vi "Get Line Colour.vi"(8 "Error In":errorcluster, 9 "Session In":T2="cam0") -> (0 "Error Out":errorcluster, 1 "Session Out":T2="cam0", 2 "Confidence (0-100)":dbl=99.96947916666667, 3 "Colour":T3=enum."None", 5 "Blue":dbl=0.030520833333333334)   [LabVIEW 2017]
uses:
  Colour Typedef 2.ctl
  <vilib>/userdefined/High Color/IMAQdx.ctl
  Globals/Pose.vi
  <vilib>/vision/NI_Vision_Development_Module.lvlib
panel:
  out "White":dbl
  in  "White Definition":T1={"Hue Range"={"Lower value"=0, "Upper value"=30}, "Saturation Range"={"Lower value"=0, "Upper value"=30}, "Luminosity Range"={"Lower value"=190, "Upper value"=230}}
  in  "Yellow Threshold":dbl=0.22
  in  "Blue Definition":T1={"Hue Range"={"Lower value"=145, "Upper value"=175}, "Saturation Range"={"Lower value"=10, "Upper value"=70}, "Luminosity Range"={"Lower value"=30, "Upper value"=115}}
  out "Yellow":dbl
  out "Red":dbl
  out "Black":dbl=0.012083333333333333
  out "Green":dbl
  in  "Threshold":dbl=0.15
  in  "Black Definition":T1={"Hue Range"={"Lower value"=0, "Upper value"=255}, "Saturation Range"={"Lower value"=0, "Upper value"=255}, "Luminosity Range"={"Lower value"=0, "Upper value"=70}}
  in  "Green Definition":T1={"Hue Range"={"Lower value"=70, "Upper value"=100}, "Saturation Range"={"Lower value"=40, "Upper value"=70}, "Luminosity Range"={"Lower value"=60, "Upper value"=95}}
  in  "Red Definition":T1={"Hue Range"={"Lower value"=0, "Upper value"=20}, "Saturation Range"={"Lower value"=80, "Upper value"=255}, "Luminosity Range"={"Lower value"=40, "Upper value"=200}}
  in  "Yellow Definition":T1={"Hue Range"={"Lower value"=10, "Upper value"=40}, "Saturation Range"={"Lower value"=80, "Upper value"=255}, "Luminosity Range"={"Lower value"=140, "Upper value"=255}}
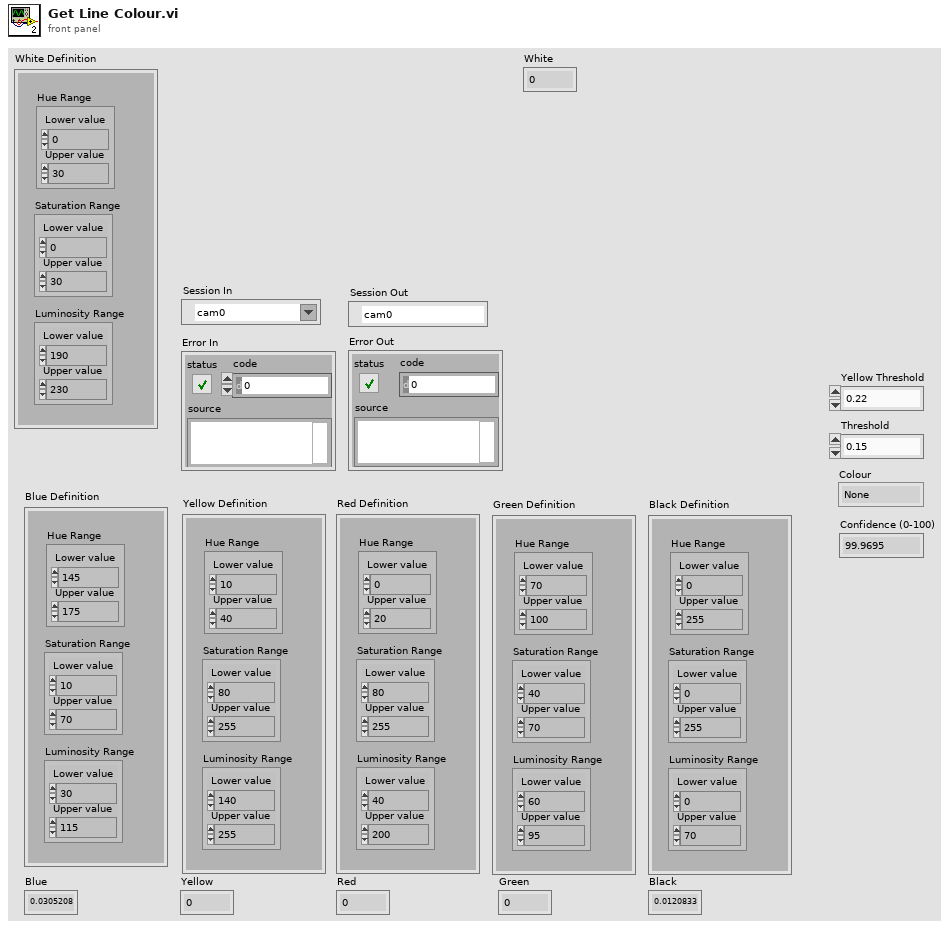
[diagram p1: front panel]
types:
  T1 = cluster{"Hue Range":cluster{"Lower value":i32, "Upper value":i32}, "Saturation Range":cluster{"Lower value":i32, "Upper value":i32}, "Luminosity Range":cluster{"Lower value":i32, "Upper value":i32}}
  T2 = typedef "IMAQdx.ctl" = refnum<k21>
  T3 = typedef "Colour Typedef 2.ctl" = enum16{"Yellow", "Black", "Green", "Blue", "None", "Black&Yellow", "Red&White"}
  T4 = typedef "Image Type" = u32
  T5 = typedef "IMAQ Image.ctl" = refnum<image>
  T6 = cluster{"Proportion":dbl, "Proportion":dbl, dbl, "Proportion":dbl}
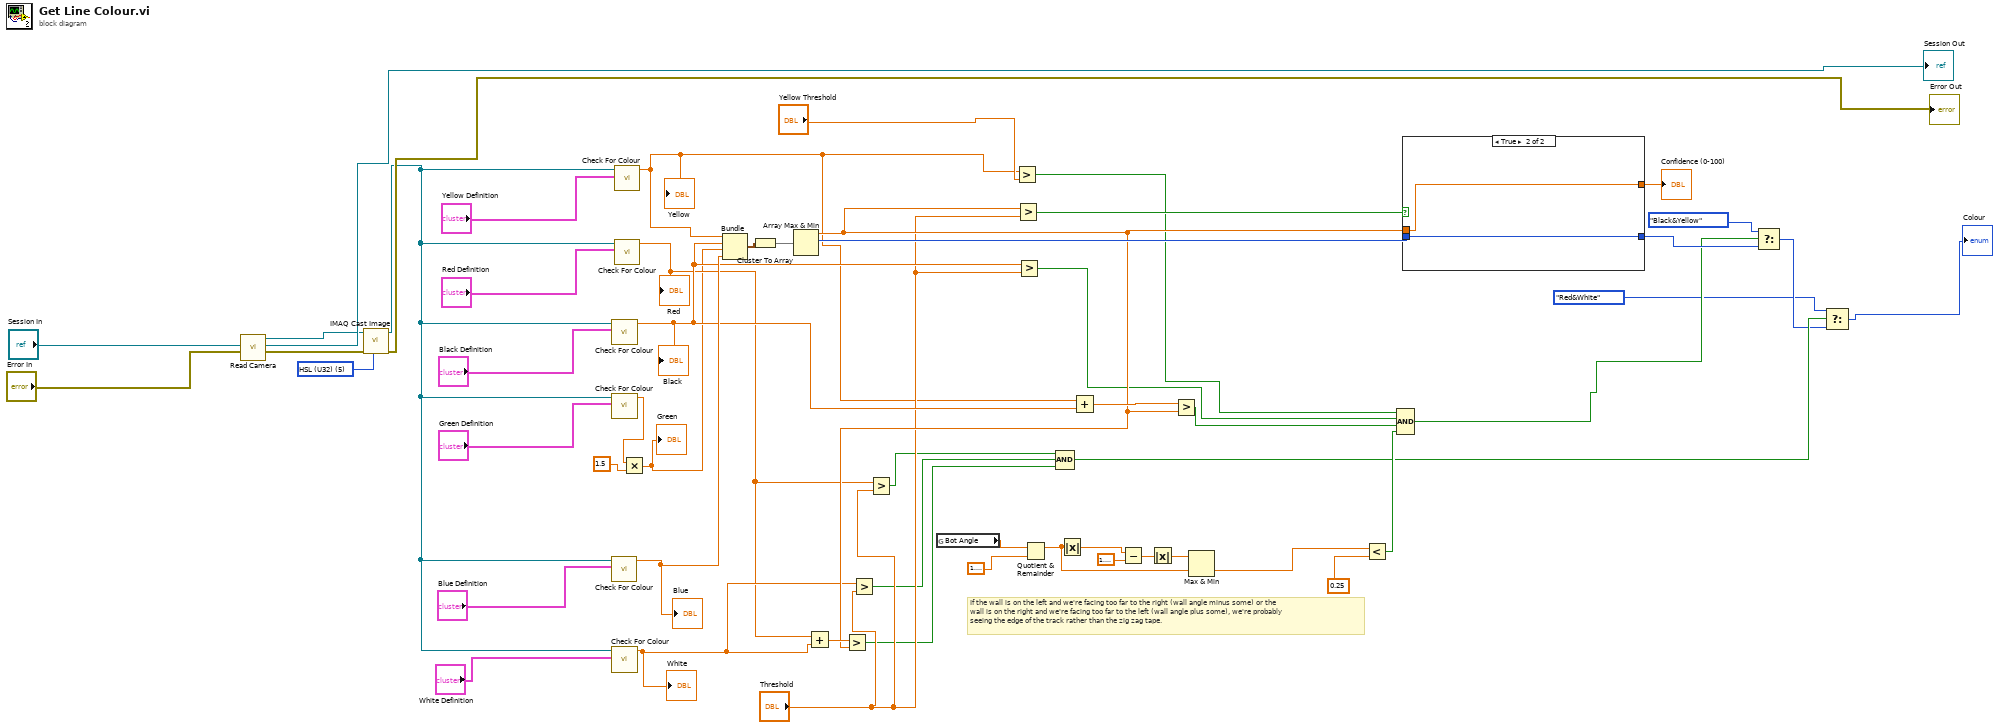
[diagram p0: block diagram]
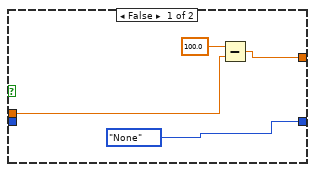
[diagram p2: hidden frame]
diagram:
  w49 = T4 5 items=["Grayscale (U8)", "Grayscale (I16)", "Grayscale (SGL)", "Complex (CSG)", "RGB (U32)", "HSL (U32)", "RGB (U64)", "Grayscale (U16)"] ("Image Type")
  # "If the wall is on the left and we're facing too far to the right (wall angle minus some) or the \nwall is on the right and we're facing too far to the left (wall angle plus some), we're probably\nseeing the edge of the track rather than the zig zag tape."
  n1 = call "Read Camera.vi"("error in"="Error In", "Session In"="Session In") -> ("error out"=w50:errorcluster, "Session Out"=→"Session Out":T2, "Image Out"=w51:T5)  [unwired: 6 in, 1 out]
  n2 = call "IMAQ Cast Image"("Image Type"=w49, "error in (no error)"=w50, "Image Src"=w51) -> ("error out"=→"Error Out":errorcluster, "Image Dst Out"=w24:T5)  [unwired: 7 in]
  n3 = call "Check For Colour.vi"("Image"=w24, "Colour Definition"="Blue Definition") -> ("Proportion"=w38:dbl)  [unwired: 8 in]
  "Blue" <- w38
  n4 = call "Check For Colour.vi"("Image"=w24, "Colour Definition"="Black Definition") -> ("Proportion"=w27:dbl)  [unwired: 8 in]
  "Black" <- w27
  n5 = call "Check For Colour.vi"("Image"=w24, "Colour Definition"="Green Definition") -> ("Proportion"=w3:dbl)  [unwired: 8 in]
  n6 = call "Check For Colour.vi"("Image"=w24, "Colour Definition"="White Definition") -> ("Proportion"=w15:dbl)  [unwired: 8 in]
  "White" <- w15
  n7 = call "Check For Colour.vi"("Image"=w24, "Colour Definition"="Yellow Definition") -> ("Proportion"=w6:dbl)  [unwired: 8 in]
  "Yellow" <- w6
  n8 = call "Check For Colour.vi"("Image"=w24, "Colour Definition"="Red Definition") -> ("Proportion"=w14:dbl)  [unwired: 8 in]
  "Red" <- w14
  n9 = Multiply(x=w3, y=1.5) -> (x*y=w1:dbl)
  "Green" <- w1
  n10 = Bundle("Proportion"=w6, "Proportion"=w27, w1, "Proportion"=w38) -> (w40:T6)  [unwired: 1 in]
  n11 = Cluster To Array(cluster=w40) -> (array=w41:dbl[])
  n12 = Array Max & Min(array=w41) -> (max value=w21:dbl, max index (indices)=w42:i32)  [unwired: 2 out]
  n13 = Add(x=w14, y=w15) -> (x+y=w22:dbl)
  n14 = Greater?(x=w22, y=w21) -> (0:w10:bool)
  n15 = Greater?(x=w15, y="Threshold") -> (0:w11:bool)
  n16 = Greater?(x=w14, y="Threshold") -> (0:w12:bool)
  n17 = global read "Pose.vi" "Bot Angle"() -> (w36:dbl)
  n18 = Greater?(x=w6, y="Yellow Threshold") -> (0:w20:bool)
  n19 = Greater?(x=w21, y="Threshold") -> (0:w44:bool)
  n20 = Greater?(x=w27, y="Threshold") -> (0:w19:bool)
  n21 = Quotient & Remainder(x=w36, y=1.5707963267948966) -> (x-y*floor(x/y)=w30:dbl)  [unwired: 1 out]
  n22 = Compound Arithmetic op=AND(w12, w11, w10) -> (w9:bool)
  n23 = Absolute Value(x=w30) -> (abs(x)=w33:dbl)
  n24 = Add(x=w6, y=w27) -> (x+y=w37:dbl)
  n25 = Subtract(x=w33, y=1.5707963267948966) -> (x-y=w32:dbl)
  n26 = Absolute Value(x=w32) -> (abs(x)=w31:dbl)
  n27 = Greater?(x=w37, y=w21) -> (0:w18:bool)
  n28 = Max & Min(x=w31, y=w30) -> (min(x,y)=w28:dbl)  [unwired: 1 out]
  n29 = Less?(x=w28, y=0.25) -> (x < y?=w17:bool)
  n30 = Compound Arithmetic op=AND(w20, w19, w18, w17) -> (w16:bool)
  n31 = case shown="True" w44 {
    tunnel: w42 -> [_ w60]
    tunnel: w21 -> [w58 w61]
    tunnel: [w57 w61] -> w43
    tunnel: [Colour_Typedef_2."None" ("Colour") w60] -> w25
    frame False {
      n32 = Subtract(x=100.0, y=w58) -> (x-y=w57:dbl)
    }
    frame True {
    }
  }
  "Confidence (0-100)" <- w43
  n33 = Select(t=Colour_Typedef_2."Black&Yellow" ("Colour"), s=w16, f=w25) -> (s? t:f=w8:i32)
  n34 = Select(t=Colour_Typedef_2."Red&White" ("Colour"), s=w9, f=w8) -> (s? t:f=→"Colour":i32)
